vi "Read (Multiple Points).vi"(8 "error in (no error)":errorcluster, 9 "Maximum Time (10000 ms)":u32=10000, 10 "Sample Count (1)":i32=1, 11 "VISA resource name":refnum<visa-resource-name>) -> (0 "error out":errorcluster, 2 "Measurements":dbl[](array[numeric]), 3 "VISA resource name out":refnum<visa-resource-name>)   [LabVIEW 2016, in "Agilent 34401.lvlib"]
doc: "Reads and returns multiple measurements from the instrument. Use this VI when you want to take multiple measurements using an immediate trigger. Use the low level VIs for other triggering options."
uses:
  <instrlib>/Agilent 34401/Agilent 34401.lvlib
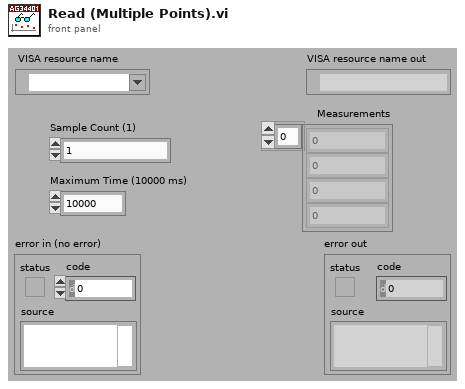
[diagram p1: front panel]
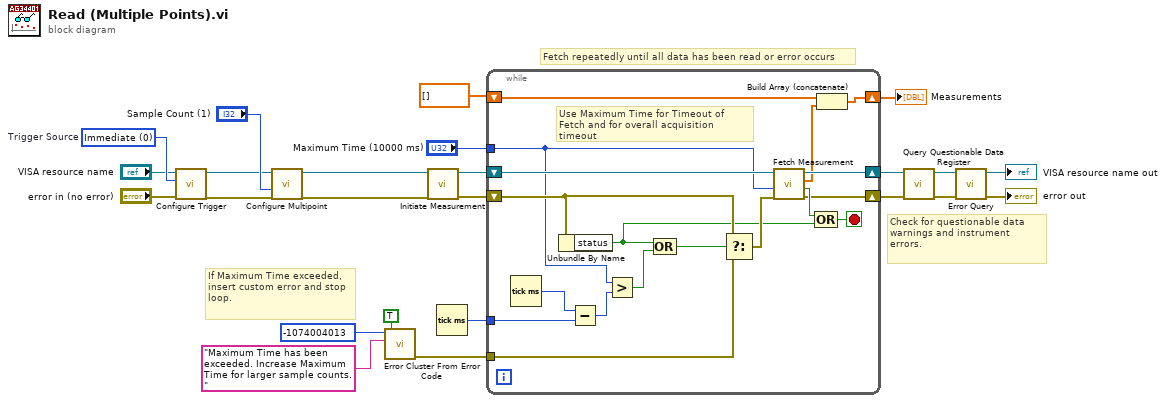
[diagram p0: block diagram]
diagram:
  w14 = u16 0 items=["Immediate", "Software (Bus)", "External", "Internal"]  # Trigger Source
  # "Check for questionable data warnings and instrument errors."
  # "If Maximum Time exceeded, insert custom error and stop loop."
  # "Fetch repeatedly until all data has been read or error occurs"
  n1 = call <instrlib>:"Configure Trigger.vi"("error in (no error)"="error in (no error)", "Trigger Source (0: Immediate)"=w14, "VISA resource name"="VISA resource name") -> ("error out"=w17:errorcluster, "VISA resource name out"=w18:refnum<visa-resource-name>)  [unwired: 7 in]
  n2 = call <instrlib>:"Configure Multipoint.vi"("error in (no error)"=w17, "Sample Count (1)"="Sample Count (1)", "VISA resource name"=w18) -> ("error out"=w15:errorcluster, "VISA resource name out"=w16:refnum<visa-resource-name>)  [unwired: 7 in]
  n3 = call <vilib>:"Error Cluster From Error Code.vi"("show call chain? (False)"=TRUE, "error message (\"\")"="Maximum Time has been exceeded. Increase Maximum Time for larger sample counts." ("Source (VI Name)"), "error code (0)"=-1074004013 ("Code")) -> ("error out"=w5:errorcluster)  [unwired: 6 in]
  n4 = call <instrlib>:"Initiate Measurement.vi"("error in (no error)"=w15, "VISA resource name"=w16) -> ("error out"=w20:errorcluster, "VISA resource name out"=w19:refnum<visa-resource-name>)  [unwired: 8 in]
  n5 = Tick Count (ms)() -> (millisecond timer value=w11:u32)
  n6 = while {
    tunnel: "Maximum Time (10000 ms)" -> [w26]
    shift-right: [w39] -> w13
    shift-left: dbl[] [] -> [w38]
    shift-right: [w42] -> w2
    shift-left: w19 -> [w41]
    shift-right: [w28] -> w1
    shift-left: w20 -> [w30]
    tunnel: w11 -> [w34]
    tunnel: w5 -> [w25]
    stop <- w36 stop-if-true
    # "Use Maximum Time for Timeout of Fetch and for overall acquisition timeout"
    n7 = Tick Count (ms)() -> (millisecond timer value=w35:u32)
    n8 = Unbundle By Name(w30) -> ("status"=w27:bool)
    n9 = Subtract(x=w35, y=w34) -> (x-y=w33:u32)
    n10 = Greater?(x=w26, y=w33) -> (0:w32:bool)
    n11 = Compound Arithmetic op=OR(w27, w32) -> (w31:bool)
    n12 = Select(t=w30, s=w31, f=w25) -> (s? t:f=w29:errorcluster)
    n13 = call <instrlib>:"Fetch Measurement.vi"("error in (no error)"=w29, "Timeout (10000 ms)"=w26, "VISA resource name"=w41) -> ("error out"=w28:errorcluster, "End of Data?"=w37:bool, "Measurements"=w40:dbl[], "VISA resource name out"=w42:refnum<visa-resource-name>)  [unwired: 5 in]
    n14 = Compound Arithmetic op=OR(w37, w27) -> (w36:bool)
    n15 = Build Array (concatenate)(w38, w40) -> (w39:dbl[])
  }
  "Measurements" <- w13
  n16 = call <instrlib>:"Query Questionable Data Register.vi"("error in (no error)"=w1, "VISA resource name"=w2) -> ("error out"=w4:errorcluster, "VISA resource name out"=w3:refnum<visa-resource-name>)  [unwired: 7 in, 1 out]
  n17 = call <instrlib>:"Error Query.vi"("error in (no error)"=w4, "VISA resource name"=w3) -> ("error out"=→"error out":errorcluster, "VISA resource name out"=→"VISA resource name out":refnum<visa-resource-name>)  [unwired: 6 in, 2 out]
